vi "Run Mazes.vi"(9 "Status Notifier":refnum<notifier>, 10 "Mouse":refnum<class "Mouse.lvclass">, 11 "Mazes":refnum<class "Maze.lvclass">[](array[class])) -> (0 "error out":errorcluster, 2 "Test Summary":string, 3 "Score":T1)   [LabVIEW 2020]
uses:
  Maze/Maze.lvclass
  Mouse/Mouse.lvclass
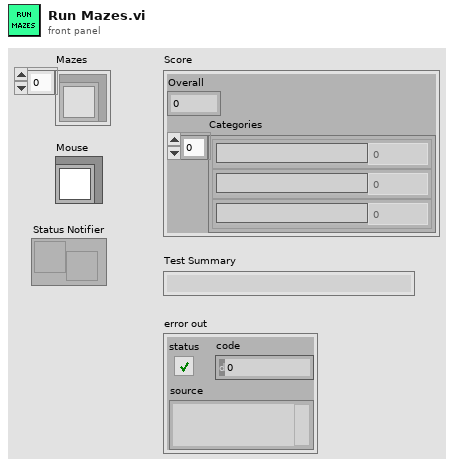
[diagram p1: front panel]
types:
  T1 = cluster{"Overall":dbl, "Categories":cluster{"Category":string, "Value":dbl}[]}
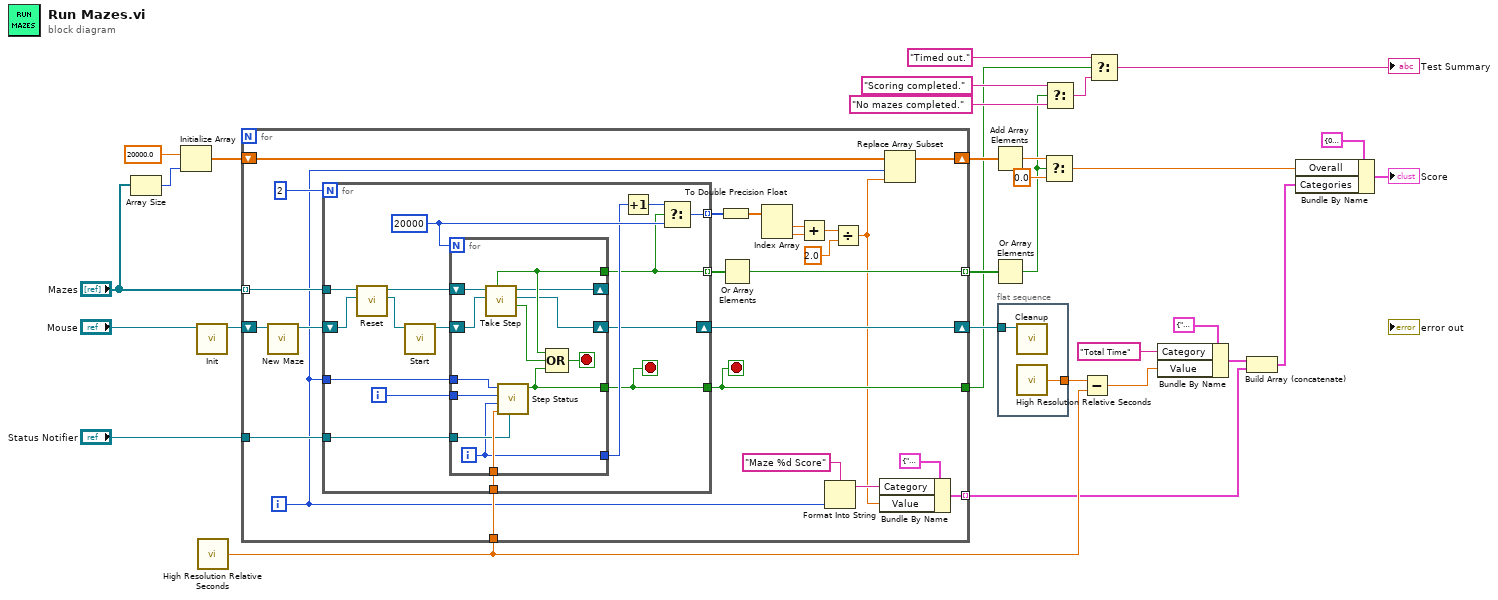
[diagram p0: block diagram]
diagram:
  n1 = Array Size(array="Mazes") -> (size(s)=w10:i32)
  n2 = Initialize Array(20000.0 ("element"), w10) -> (w8:dbl[])
  n3 = call-dynamic "Init.vi"("Mouse in"="Mouse") -> ("Mouse out"=w28:refnum<class "Mouse.lvclass">)  [unwired: 9 in, 1 out]
  n4 = call <vilib>:"High Resolution Relative Seconds.vi"() -> ("relative seconds"=w25:dbl)
  n5 = for {
    tunnel: "Mazes" -> [w53] mode=indexing
    tunnel: "Status Notifier" -> [w49]
    shift-right: [w42] -> w27
    shift-left: w28 -> [w54]
    tunnel: w25 -> [w50]
    tunnel: [w40] -> w24 mode=indexing
    tunnel: [w36] -> w14 mode=indexing
    tunnel: [w35] -> w3
    shift-right: [w33] -> w7
    shift-left: w8 -> [w34]
    i -> [w32]
    stop <- w35 stop-if-true
    n6 = call-dynamic "New Maze.vi"("Mouse in"=w54) -> ("Mouse out"=w51:refnum<class "Mouse.lvclass">)  [unwired: 9 in, 1 out]
    n7 = for {
      N: 2 -> [_]
      tunnel: w53 -> [w70]
      tunnel: w50 -> [w67]
      shift-right: [w57] -> w42
      shift-left: w51 -> [w69]
      tunnel: w49 -> [w64]
      tunnel: w32 -> [w62]
      tunnel: [w58] -> w48 mode=indexing
      tunnel: [w56] -> w41 mode=indexing
      tunnel: [w55] -> w35
      i -> [w63]
      stop <- w55 stop-if-true
      w61 = 20000
      n8 = call "Reset.vi"("Mouse In"=w69, "Maze in"=w70) -> ("Mouse"=w68:refnum<class "Mouse.lvclass">, "Maze out"=w66:refnum<class "Maze.lvclass">)  [unwired: 7 in, 1 out]
      n9 = call-dynamic "Start.vi"("Mouse in"=w68) -> ("Mouse out"=w65:refnum<class "Mouse.lvclass">)  [unwired: 9 in, 1 out]
      n10 = for {
        N: w61 -> [_]
        tunnel: w67 -> [w77]
        shift-right: [w79] -> _
        shift-left: w66 -> [w83]
        shift-right: [w78] -> w57
        shift-left: w65 -> [w82]
        tunnel: [w80] -> w56
        tunnel: [w75] -> w60
        tunnel: w64 -> [w76]
        tunnel: w63 -> [w74]
        tunnel: w62 -> [w73]
        tunnel: [w71] -> w55
        i -> [w75]
        stop <- w81 stop-if-true
        n11 = call "Take Step.vi"("Mouse In"=w82, "Maze in"=w83) -> ("Bad Action?"=w72:bool, "Mouse"=w78:refnum<class "Mouse.lvclass">, "Maze"=w79:refnum<class "Maze.lvclass">, "Goal?"=w80:bool)  [unwired: 2 in, 4 out]
        n12 = call "Step Status.vi"("Status Notifier"=w76, "Start Time"=w77, "Action"=w75, "Run"=w74, "Maze"=w73) -> ("Timeout?"=w71:bool)  [unwired: 6 in]
        n13 = Compound Arithmetic op=OR(w80, w72, w71) -> (w81:bool)
      }
      n14 = Increment(x=w60) -> (x+1=w59:i32)
      n15 = Select(t=w59, s=w56, f=w61) -> (s? t:f=w58:i32)
    }
    n16 = To Double Precision Float(number=w48) -> (double precision float=w47:dbl[])
    n17 = Or Array Elements(Boolean array=w41) -> (logical OR=w40:bool)
    n18 = Index Array(array=w47) -> (element #1=w46:dbl, element #2=w45:dbl)  [unwired: 2 in]
    n19 = Add(x=w46, y=w45) -> (x+y=w44:dbl)
    n20 = Format Into String(format string="Maze %d Score", w32) -> (resulting string=w38:string)  [unwired: 2 in, 1 out]
    n21 = Divide(x=w44, y=2.0) -> (x/y=w31:dbl)
    n22 = Bundle By Name(cluster=cluster{"Category":string, "Value":dbl} {"Category"="", "Value"=0.0} ("Score Entry"), "Category"=w38, "Value"=w31) -> (w36:cluster{"Category":string, "Value":dbl})
    n23 = Replace Array Subset(array=w34, new element=w31, index=w32) -> (w33:dbl[])
  }
  n24 = Add Array Elements(numeric array=w7) -> (sum=w21:dbl)
  n25 = Or Array Elements(Boolean array=w24) -> (logical OR=w5:bool)
  n26 = flat-sequence {
    tunnel: w27 -> [w85]
    tunnel: [w84] -> w26
    frame #0 {
      n27 = call-dynamic "Cleanup.vi"("Mouse in"=w85) -> ()  [unwired: 10 in, 1 out]
      n28 = call <vilib>:"High Resolution Relative Seconds.vi"() -> ("relative seconds"=w84:dbl)
    }
  }
  n29 = Select(t=w21, s=w5, f=0.0) -> (s? t:f=w19:dbl)
  n30 = Select(t="Scoring completed.", s=w5, f="No mazes completed.") -> (s? t:f=w2:string)
  n31 = Subtract(x=w26, y=w25) -> (x-y=w17:dbl)
  n32 = Select(t="Timed out.", s=w3, f=w2) -> (s? t:f=→"Test Summary":string)
  n33 = Bundle By Name(cluster=cluster{"Category":string, "Value":dbl} {"Category"="", "Value"=0.0} ("Score Entry"), "Category"="Total Time", "Value"=w17) -> (w15:cluster{"Category":string, "Value":dbl})
  n34 = Build Array (concatenate)(w15, w14) -> (w13:cluster{"Category":string, "Value":dbl}[])
  n35 = Bundle By Name(cluster=T1 {"Overall"=0.0, "Categories"=[]} ("Score"), "Overall"=w19, "Categories"=w13) -> (→"Score":T1)
